vi "Thermistor_Conversion.vi"(10 "Voltage Readings":dbl[](array[numeric]), 11 "DataCluster":T1={"Core"={"Current VI Reference"=refnum, "Close Panel on Exit?"=FALSE, "Exit"=FALSE}, "Connections"={"cDAQ Therm"={"Task"="", "Connected"=FALSE, "Active"=FALSE}, "cDAQ Voltage"={"Task"="", "Connected"=FALSE, "Active"=FALSE}, "cDAQ ID"="", "Camera"={"Session"="", "Connected"=FALSE, "Active"=FALSE}}, "Data Acquisition"={"Setup"={"Label"="", "Operator"="", "Notes"="", "TempGrad"=1.0, "TargetTemp"=1.0, "Sample Volume"=1.0}, "Camera"={"Image"=refnum, "Save Image"=refnum, "Image Frequency"=20, "Rectangle"={"Left"=0, "Top"=0, "Right"=0, "Bottom"=0, "Rotation"=0.0}}, "Thermistor"={"Sample Size"=1, "Calibration"={"B0.100"=[], "R25"=[], "c"=[], "State"=[], "V_S"=5.0, "R_S"=100.0}, "Timing Mode"=14713}, "Partition"={"Data"=[], "Cell Label"="", "Cell Color"=0, "Height"=10, "Width"=16, "Grid"=[]}, "Queue"={"Queue"=refnum, "Size"=1}, "Sample Rate"=1, "Active"=FALSE, "Ready"=FALSE, "Graph Mode"=0}, "Control"={"Sample Rate"=1, "PID gains"={"proportional gain (Kc)"=1.0, "integral time (Ti, min)"=0.01, "derivative time (Td, min)"=0.0}}} {"Control"."PID gains"."derivative time (Td, min)" format="%.3f"; "Control"."PID gains"."integral time (Ti, min)" format="%.3f"; "Control"."PID gains"."proportional gain (Kc)" format="%.3f"; "Control"."Sample Rate" min=1 max=20 step=1 format="%.0f Samples/sec"; "Data Acquisition"."Graph Mode" items=["Average Temperature", "Individual Temperatures"]; "Data Acquisition"."Thermistor"."Timing Mode" items=["Automatic"=16097, "High Resolution"=10195, "High Speed"=14712, "Best 50 Hz Rejection"=14713, "Best 60 Hz Rejection"=14714, "Custom"=10137]; "Data Acquisition"."Thermistor"."Calibration"."R_S" min=0.1 max=1000.0 format="%#_g kOhm"; "Data Acquisition"."Thermistor"."Calibration"."V_S" min=5.0 max=48.0 format="%#_g V"; "Data Acquisition"."Thermistor"."Calibration"."R25" min=0.1 max=1000.0 format="%#_g kOhm"; "Data Acquisition"."Thermistor"."Calibration"."B0.100" min=100.0 max=10000.0 format="%#_g K"; "Data Acquisition"."Thermistor"."Sample Size" min=1 max=200; "Data Acquisition"."Sample Rate" min=20 max=240 format="%.0f samples/min"; "Data Acquisition"."Queue"."Size" min=1 max=200; "Data Acquisition"."Camera"."Rectangle"."Rotation" min=-90.0 max=90.0 step=1.0 format="%.2f"; "Data Acquisition"."Camera"."Rectangle"."Left" scale=0.0..1024.0; "Data Acquisition"."Camera"."Rectangle"."Right" scale=0.0..1024.0; "Data Acquisition"."Camera"."Image Frequency" min=1 max=60 step=1; "Data Acquisition"."Setup"."Sample Volume" min=0.0 max=500.0 format="%#_g µL"; "Data Acquisition"."Setup"."TargetTemp" min=-40.0 max=40.0 step=0.5 format="%#_g °C"; "Data Acquisition"."Setup"."TempGrad" min=-100.0 max=100.0 step=0.1 format="%#_g °C/min"}) -> (1 "Mean Temp":dbl format="%0.2f", 2 "Temperature Readings":dbl[](array[numeric]))   [LabVIEW 2020]
uses:
  DataCluster.ctl
  <vilib>/userDefined/High Color/IMAQdx.ctl
  <vilib>/vision/Image Controls.llb/IMAQ Image.ctl
  <vilib>/Analysis/baseanly.llb/Mean (DBL).vi
  <vilib>/Analysis/NI_AALBase.lvlib
panel:
  out "Data Acquisition.Thermistor.Calibration.State":bool[](array[boolean])
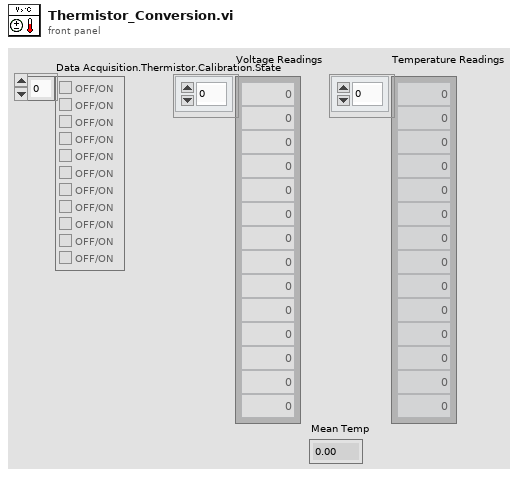
[diagram p1: front panel]
types:
  T1 = typedef "DataCluster.ctl" = cluster{"Core":cluster{"Current VI Reference":refnum<vi>, "Close Panel on Exit?":bool, "Exit":bool}, "Connections":cluster{"cDAQ Therm":cluster{"Task":refnum<k21>, "Connected":bool, "Active":bool}, "cDAQ Voltage":cluster{"Task":refnum<k21>, "Connected":bool, "Active":bool}, "cDAQ ID":string, "Camera":cluster{"Session":T2, "Connected":bool, "Active":bool}}, "Data Acquisition":cluster{"Setup":cluster{"Label":string, "Operator":string, "Notes":string, "TempGrad":dbl, "TargetTemp":dbl, "Sample Volume":dbl}, "Camera":cluster{"Image":T3, "Save Image":T3, "Image Frequency":i32, "Rectangle":T4}, "Thermistor":cluster{"Sample Size":i32, "Calibration":cluster{"B0.100":dbl[], "R25":dbl[], "c":dbl[][], "State":bool[], "V_S":dbl, "R_S":dbl}, "Timing Mode":i32}, "Partition":cluster{"Data":string[][], "Cell Label":string, "Cell Color":u32, "Height":i32, "Width":i32, "Grid":string[][]}, "Queue":cluster{"Queue":refnum<queue>, "Size":i32}, "Sample Rate":i32, "Active":bool, "Ready":bool, "Graph Mode":u16}, "Control":cluster{"Sample Rate":i32, "PID gains":cluster{"proportional gain (Kc)":dbl, "integral time (Ti, min)":dbl, "derivative time (Td, min)":dbl}}}
  T2 = typedef "IMAQdx.ctl" = refnum<k21>
  T3 = typedef "IMAQ Image.ctl" = refnum<image>
  T4 = typedef "IMAQ Rectangle" = cluster{"Left":i32, "Top":i32, "Right":i32, "Bottom":i32, "Rotation":dbl}
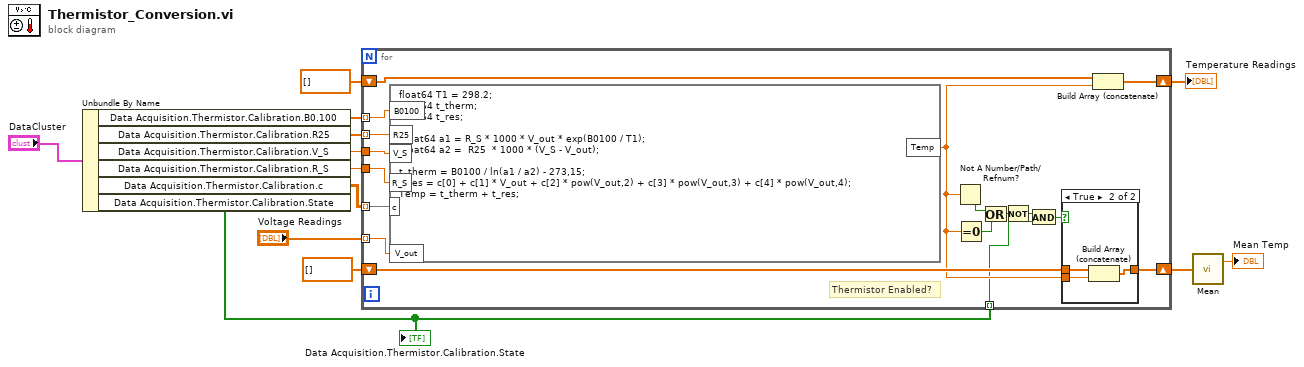
[diagram p0: block diagram]
diagram:
  n1 = Unbundle By Name("DataCluster") -> ("Data Acquisition.Thermistor.Calibration.B0.100"=w12:dbl[], "Data Acquisition.Thermistor.Calibration.R25"=w11:dbl[], "Data Acquisition.Thermistor.Calibration.V_S"=w9:dbl, "Data Acquisition.Thermistor.Calibration.R_S"=w8:dbl, "Data Acquisition.Thermistor.Calibration.c"=w2:dbl[][], "Data Acquisition.Thermistor.Calibration.State"=w1:bool[])
  "Data Acquisition.Thermistor.Calibration.State" <- w1
  n2 = for {
    tunnel: w12 -> [w30] mode=indexing
    tunnel: w11 -> [w29] mode=indexing
    tunnel: "Voltage Readings" -> [w28] mode=indexing
    tunnel: w9 -> [w27]
    tunnel: w8 -> [w26]
    shift-right: [w25] -> w6
    shift-left: dbl[] [] -> [w24]
    shift-right: [w22] -> w4
    shift-left: dbl[] [] -> [w21]
    tunnel: w2 -> [w18] mode=indexing
    tunnel: w1 -> [w16] mode=indexing
    # "Thermistor Enabled?"
    n3 = formula code="float64 T1 = 298.2;\nfloat64 t_therm;\nfloat64 t_res;\n\n float64 a1 = R_S * 1000 * V_out * exp(B0100 / T1);\n float64 a2 =  R25  * 1000 * (V_S - V_out);\n\nt_therm = B0100 / ln(a1 / a2) - 273,15;\nt_res = c[0] + c[1] * V_out + c[2] * pow(V_out,2) + c[3] * pow(V_out,3) + c[4] * pow(V_out,4);\nTemp = t_therm + t_res;"("B0100"=w30, "R25"=w29, "V_out"=w28, "V_S"=w27, "R_S"=w26, "c"=w18) -> ("Temp"=w19:dbl)
    n4 = Not A Number/Path/Refnum?(number/path/refnum=w19) -> (NaN/Path/Refnum?=w23:bool)
    n5 = Equal To 0?(x=w19) -> (x = 0?=w20:bool)
    n6 = Or(x=w23, y=w20) -> (x .or. y?=w15:bool)
    n7 = Not(x=w15) -> (.not. x?=w14:bool)
    n8 = And(x=w14, y=w16) -> (x .and. y?=w17:bool)
    n9 = case shown="True" w17 {
      tunnel: w19 -> [_ w34]
      tunnel: [w31 w33] -> w22
      tunnel: w21 -> [w31 w32]
      frame False {
      }
      frame True {
        n10 = Build Array (concatenate)(w32, w34) -> (w33:dbl[])
      }
    }
    n11 = Build Array (concatenate)(w24, w19) -> (w25:dbl[])
  }
  "Temperature Readings" <- w6
  n12 = call-poly <vilib>:"Mean.vi"("X"=w4) -> ("mean"=→"Mean Temp":dbl)  [unwired: 1 out]
